vi "EN1 VIs.vi"() -> ()   [LabVIEW 2019]
uses:
  <vilib>/httpClient/LabVIEWHTTPClient.lvlib
  <vilib>/httpClient/POSTBuffer.vi
  <vilib>/httpClient/PUTBuffer.vi
  ThingWorx/_TW_Subs/Thingworx_Write_Bool.vi
  SystemLink/SL_Subs/SystemLink_Write_Boolean.vi
  OpenDiagram/Open_XControl.xctl
panel:
  in  "OpenDiag":refnum<vi>(xcontrol)
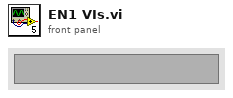
[diagram p1: front panel]
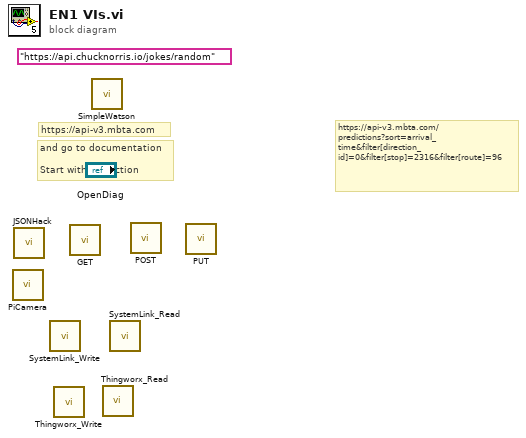
[diagram p0: block diagram]
diagram:
  (unwired) "https://api.chucknorris.io/jokes/random"
  # "https://api-v3.mbta.com/predictions?sort=arrival_time&filter[direction_id]=0&filter[stop]=2316&filter[route]=96"
  # "and go to documentation\n\nStart with prediction"
  # "https://api-v3.mbta.com"
  n1 = call "PiCamera.vi"() -> ()  [unwired: 12 in]
  n2 = call "JSONHack.vi"() -> ()  [unwired: 8 in, 4 out]
  n3 = call-poly "SystemLink_Write.vi"() -> ()  [unwired: 12 in]
  n4 = call-poly "Thingworx_Write.vi"() -> ()  [unwired: 12 in]
  n5 = call <vilib>:"GET.vi"() -> ()  [unwired: 12 in, 4 out]
  n6 = call "SimpleWatson.vi"() -> ()  [unwired: 12 in]
  n7 = call "Thingworx_Read.vi"() -> ()  [unwired: 10 in, 2 out]
  n8 = call "SystemLink_Read.vi"() -> ()  [unwired: 9 in, 3 out]
  n9 = call-poly <vilib>:"POST.vi"() -> ()  [unwired: 12 in, 4 out]
  n10 = call-poly <vilib>:"PUT.vi"() -> ()  [unwired: 12 in, 4 out]
